vi "find first peak - amplitude (SubVI).vi"(6 "Noise length":i32=5, 8 "Noise min":dbl, 9 "threshold ratio":dbl=3.0, 10 "width":i32=3, 11 "Array":dbl[](array[numeric])) -> (0 "Peak threshold":dbl, 1 "noise index":dbl[](array[numeric]), 2 "peak amplitude":dbl, 3 "Index":dbl, 4 "#peaks":i32)   [LabVIEW 2012]
uses:
  <vilib>/Analysis/NI_AAL_SigProc.lvlib
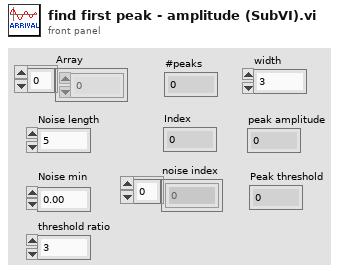
[diagram p1: front panel]
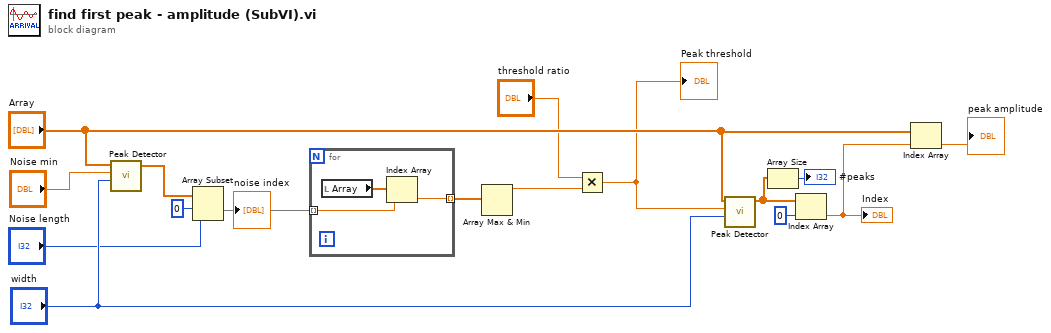
[diagram p0: block diagram]
diagram:
  n1 = call <vilib>:"Peak Detector.vi"("width"="width", "threshold"="Noise min", "X"="Array") -> ("Locations"=w9:dbl[])  [unwired: 4 in, 4 out]
  n2 = Array Subset(array=w9, index=0, length="Noise length") -> (w7:dbl[])
  "noise index" <- w7
  n3 = for {
    tunnel: w7 -> [w19] mode=indexing
    tunnel: [w17] -> w5 mode=indexing
    n4 = local read "Array"() -> (w18:dbl[])
    n5 = Index Array(array=w18, index=w19) -> (element=w17:dbl)
  }
  n6 = Array Max & Min(array=w5) -> (max value=w4:dbl)  [unwired: 3 out]
  n7 = Multiply(x="threshold ratio", y=w4) -> (x*y=w3:dbl)
  "Peak threshold" <- w3
  n8 = call <vilib>:"Peak Detector.vi"("width"="width", "threshold"=w3, "X"="Array") -> ("Locations"=w14:dbl[])  [unwired: 4 in, 4 out]
  n9 = Array Size(array=w14) -> (size(s)=→"#peaks":i32)
  n10 = Index Array(array=w14, index=0) -> (element=w13:dbl)
  "Index" <- w13
  n11 = Index Array(array="Array", index=w13) -> (element=→"peak amplitude":dbl)
